vi "FP show the boat.vi"(2 "GPS":cluster{"X pos":i32, "Y pos":i32, "Heading":dbl}, 3 "Boat array":u32[][](array[numeric]), 4 "Pool array":u32[][](array[numeric])) -> (1 "Pool out":u32[][](array[numeric]))   [LabVIEW 2014]
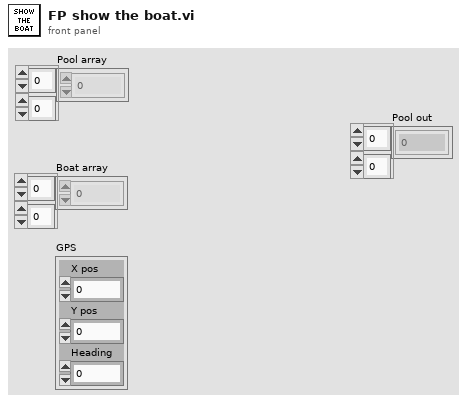
[diagram p1: front panel]
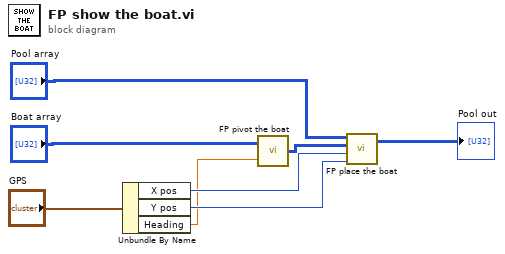
[diagram p0: block diagram]
diagram:
  n1 = Unbundle By Name("GPS") -> ("X pos"=w7:i32, "Y pos"=w6:i32, "Heading"=w5:dbl)
  n2 = call "FP pivot the boat.vi"("Heading"=w5, "Image Pixels (U32)"="Boat array") -> ("Image pixels\nOut"=w8:u32[][])
  n3 = call "FP place the boat.vi"("Y pos"=w6, "X pos"=w7, "Boat image\nPixels (U32)"=w8, "Pool image\nPixels (U32)"="Pool array") -> ("Pool image\nPixels (U32) out"=→"Pool out":u32[][])  [unwired: 1 in]
